vi "Get Item Property (Variant).vi"(8 "error in (no error)":errorcluster, 9 "Default Value":variant, 10 "Property Name":string, 11 "Item Ref in":T1 format="%.0x") -> (0 "error out":errorcluster, 1 "Value":variant, 3 "Item Ref out":T1 format="%.0x", 4 "Found?":bool)   [LabVIEW 2020, in "Custom Device Offline API.lvlib"]
uses:
  <vilib>/NI VeriStand/Custom Device Offline API/Custom Device Offline API.lvlib
  <vilib>/NI VeriStand/Custom Device API/Custom Device Item Ref.ctl
  <vilib>/NI VeriStand/Custom Device API/Custom Device API.lvlib
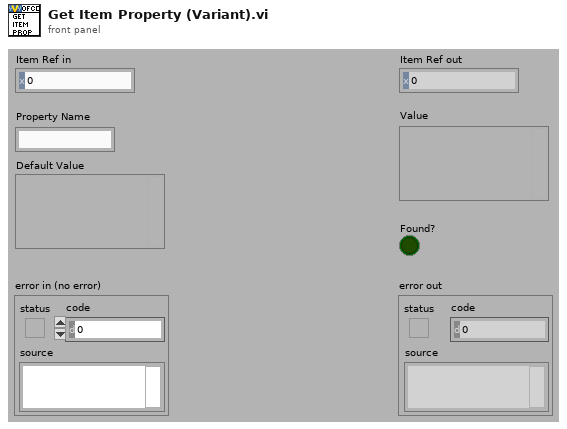
[diagram p1: front panel]
types:
  T1 = typedef "Custom Device API.lvlib/Custom Device Item Ref.ctl" = u64
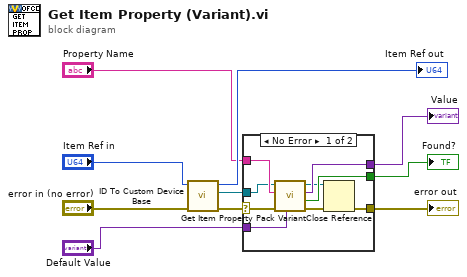
[diagram p0: block diagram]
diagram:
  n1 = call <vilib>:"ID To Custom Device Base.vi"("error in (no error)"="error in (no error)", "ID in"="Item Ref in") -> ("error out"=w5:errorcluster, "BaseNode"=w4:refnum<k24>, "ID out"=→"Item Ref out":u64)  [unwired: 7 in]
  n2 = case shown="No Error" w5 {
    selector: w5 -> [w17 w20]
    tunnel: "Default Value" -> [w19 w21]
    tunnel: "Property Name" -> [w18 _]
    tunnel: w4 -> [w16 _]
    tunnel: [w15 w21] -> w3
    tunnel: [w14 _] -> w2
    tunnel: [w11 w20] -> w1
    frame No Error {
      n3 = call <vilib>:"Get Item Property Pack Variant.vi"("Default Value"=w19, "error in (no error)"=w17, "Property Name"=w18, "CDBase"=w16) -> ("error out"=w12:errorcluster, "Found?"=w14:bool, "Variant"=w15:variant, "CDBase"=w13:refnum<k24>)  [unwired: 4 in]
      n4 = Close Reference(reference=w13, error in (no error)=w12) -> (error out=w11:errorcluster)
    }
    frame Error {
    }
  }
  "error out" <- w1
  "Value" <- w3
  "Found?" <- w2
